vi "SetSyStime.vi"() -> ()   [LabVIEW 2015]
uses:
  C:/Windows/System32/kernel32.dll
panel:
  in  "簇":T1={"年"=2018, "月"=11, "星期"=7, "日"=20, "小时"=10, "分"=10, "秒"=59, "毫秒"=800}
  out "返回类型":i8
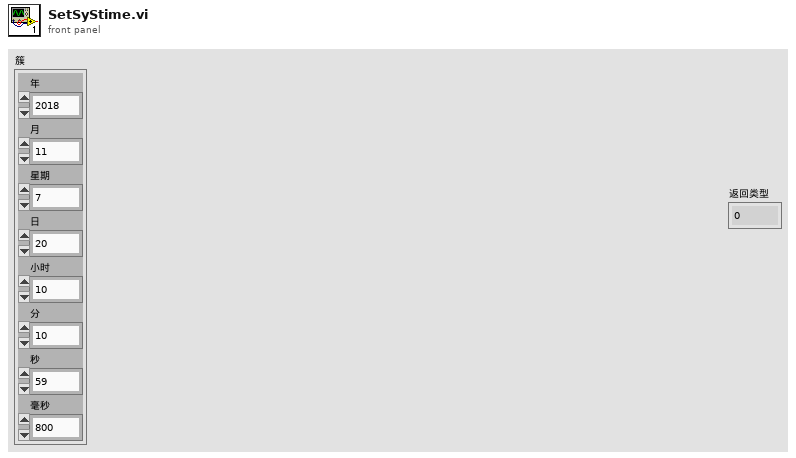
[diagram p1: front panel]
types:
  T1 = cluster{"年":u16, "月":u16, "星期":u16, "日":u16, "小时":u16, "分":u16, "秒":u16, "毫秒":u16}
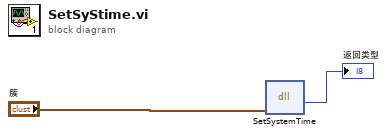
[diagram p0: block diagram]
diagram:
  n1 = dll-call lib="C:/Windows/System32/kernel32.dll" fn="SetSystemTime"("系统时间"="簇") -> ("返回类型"=→"返回类型":i8)  [unwired: 4 in, 2 out]
